vi "LCC Create PID Control Channel.vi"(7 "Control Loop Output Type":T1 items=["ANALOG", "DIGITAL", "DIGITAL_PWM", "PUMP_FLOW"], 8 "error in (no error)":errorcluster caption="Fehler (Eingang, kein Fehler)", 10 "Output":i64, 11 "AnalogInput":i64) -> (0 "error out":errorcluster caption="Fehler (Ausgang)", 3 "Control Channel":i64)   [LabVIEW 2021, in "labbCAN_Controller_API.lvlib"]
doc: "LCC_Func long LCC_CALL LCC_CreatePIDControlChannel(dev_hdl AnalogInput, dev_hdl Output,\n unsigned int LoopOutType, dev_hdl* pCreatedChannel);"
uses:
  labbCAN_Controller_API.lvlib
  LoopOutType.ctl
  labbCAN_Controller_API.dll
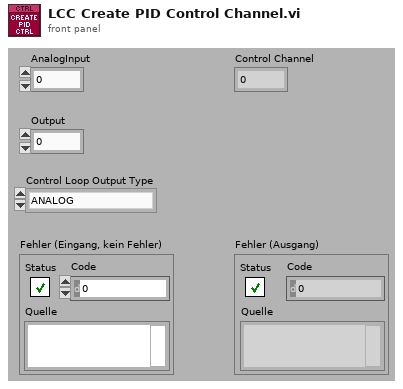
[diagram p1: front panel]
types:
  T1 = typedef "labbCAN_Controller_API.lvlib/LoopOutType.ctl" = u32
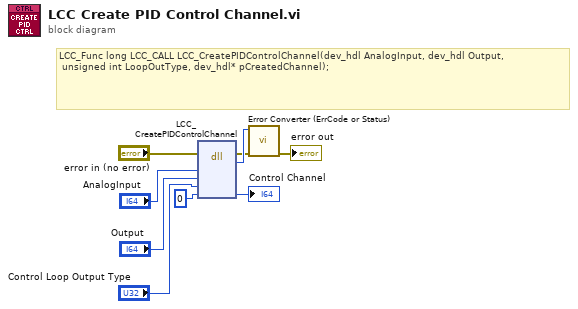
[diagram p0: block diagram]
diagram:
  # "LCC_Func long LCC_CALL LCC_CreatePIDControlChannel(dev_hdl AnalogInput, dev_hdl Output,\n\tunsigned int LoopOutType, dev_hdl* pCreatedChannel);"
  n1 = dll-call lib="C:/Users/olaja/AppData/Local/CETONI_SDK/labbCAN_Controller_API.*" fn="LCC_CreatePIDControlChannel"(error in="error in (no error)", "AnalogInput"="AnalogInput", "Output"="Output", "LoopOutType"="Control Loop Output Type", "pCreatedChannel"=i64 0) -> (error out=w3:errorcluster, "Rückgabetyp"=w4:i32, "pCreatedChannel"=→"Control Channel":i64)  [unwired: 5 in, 1 out]
  n2 = call "Error Converter (ErrCode or Status).vi"("error in (no error)"=w3, "error code"=w4) -> ("error out"=→"error out":errorcluster)  [unwired: 9 in]
